vi "Get NrOfTXPDO.vi"(11 "Device Info in":refnum<class "Device Info.lvclass">) -> (2 "NrOfTXPDO":u16, 3 "Device Info out":refnum<class "Device Info.lvclass">)   [LabVIEW 2019, in "Electronic Datasheet.lvlib" / "Device Info.lvclass"]
uses:
  Device Info.lvclass
  Device Info.lvclass/Device Info.ctl
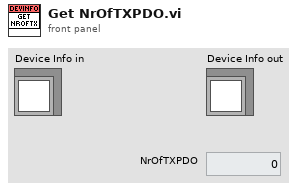
[diagram p1: front panel]
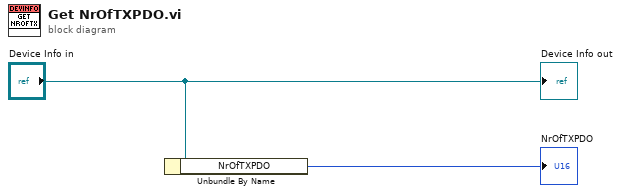
[diagram p0: block diagram]
diagram:
  n1 = Unbundle By Name("Device Info in") -> ("NrOfTXPDO"=→"NrOfTXPDO":u16)
  "Device Info out" <- "Device Info in"
